vi "VI tree.vi"   [LabVIEW 2021, in "F-70 driver.lvlib"]
uses:
  <instrlib>/F-70 driver/F-70 driver.lvlib
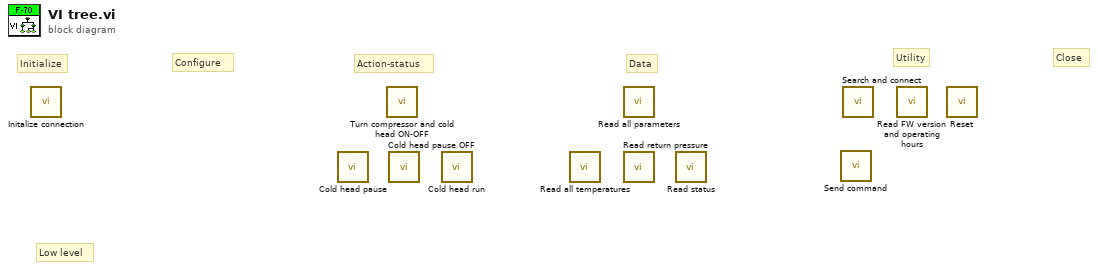
[diagram p0: block diagram]
diagram:
  # "Low level"
  # "Action-status"
  # "Close"
  # "Utility"
  # "Data"
  # "Configure"
  # "Initialize"
  n1 = call <instrlib>:"Initalize connection.vi"() -> ()  [unwired: 5 in, 3 out]
  n2 = call <instrlib>:"Cold head pause.vi"() -> ()  [unwired: 8 in, 4 out]
  n3 = call <instrlib>:"Turn compressor and cold head ON-OFF.vi"() -> ()  [unwired: 8 in, 4 out]
  n4 = call <instrlib>:"Cold head pause OFF.vi"() -> ()  [unwired: 8 in, 4 out]
  n5 = call <instrlib>:"Cold head run.vi"() -> ()  [unwired: 8 in, 4 out]
  n6 = call <instrlib>:"Read all temperatures.vi"() -> ()  [unwired: 6 in, 6 out]
  n7 = call <instrlib>:"Read all parameters.vi"() -> ()  [unwired: 5 in, 3 out]
  n8 = call <instrlib>:"Read return pressure.vi"() -> ()  [unwired: 4 in, 4 out]
  n9 = call <instrlib>:"Read status.vi"() -> ()  [unwired: 4 in, 4 out]
  n10 = call <instrlib>:"Send command.vi"() -> ()  [unwired: 5 in, 3 out]
  n11 = call <instrlib>:"Search and connect.vi"() -> ()  [unwired: 10 in, 2 out]
  n12 = call <instrlib>:"Read FW version and operating hours.vi"() -> ()  [unwired: 7 in, 5 out]
  n13 = call <instrlib>:"Reset.vi"() -> ()  [unwired: 9 in, 3 out]
